vi "Target.vi"   [LabVIEW 2025]
uses:
  <vilib>/eio/utilities/niEioResolveVilibRelativePath.vi
  <vilib>/rvi/interface/RandomDataEmulation/niFpgaRandomDataHandleErrors.vi
  <vilib>/rvi/Memory/Memory_Emulation/nirvimemoryFastEmulation.vi
  <vilib>/rvi/Memory/Memory_Emulation/nirvimemoryEmulation.vi
  <vilib>/rvi/Emulation/niFpgaEmulationIsFPGAContextNoSignature.vi
  <vilib>/rvi/DataTransferAndStorage/Container/Common/niFpgaContainerGetUniqueNameForEmu.vi
  <vilib>/rvi/Emulation/niFpgaProcessEmulError.vi
  <vilib>/rvi/Emulation/niFpgaSctlEmulationGetInTimedLoop.vi
  <vilib>/rvi/errors/nirviReportUnexpectedCaseInternalError (U32).vi
  <vilib>/rvi/DataTransferAndStorage/Container/XNode/niFpgaContainer.xnode
  <vilib>/rvi/interface/RandomDataEmulation/nirviRandomDataFpgaReadWriteTemplate.vi
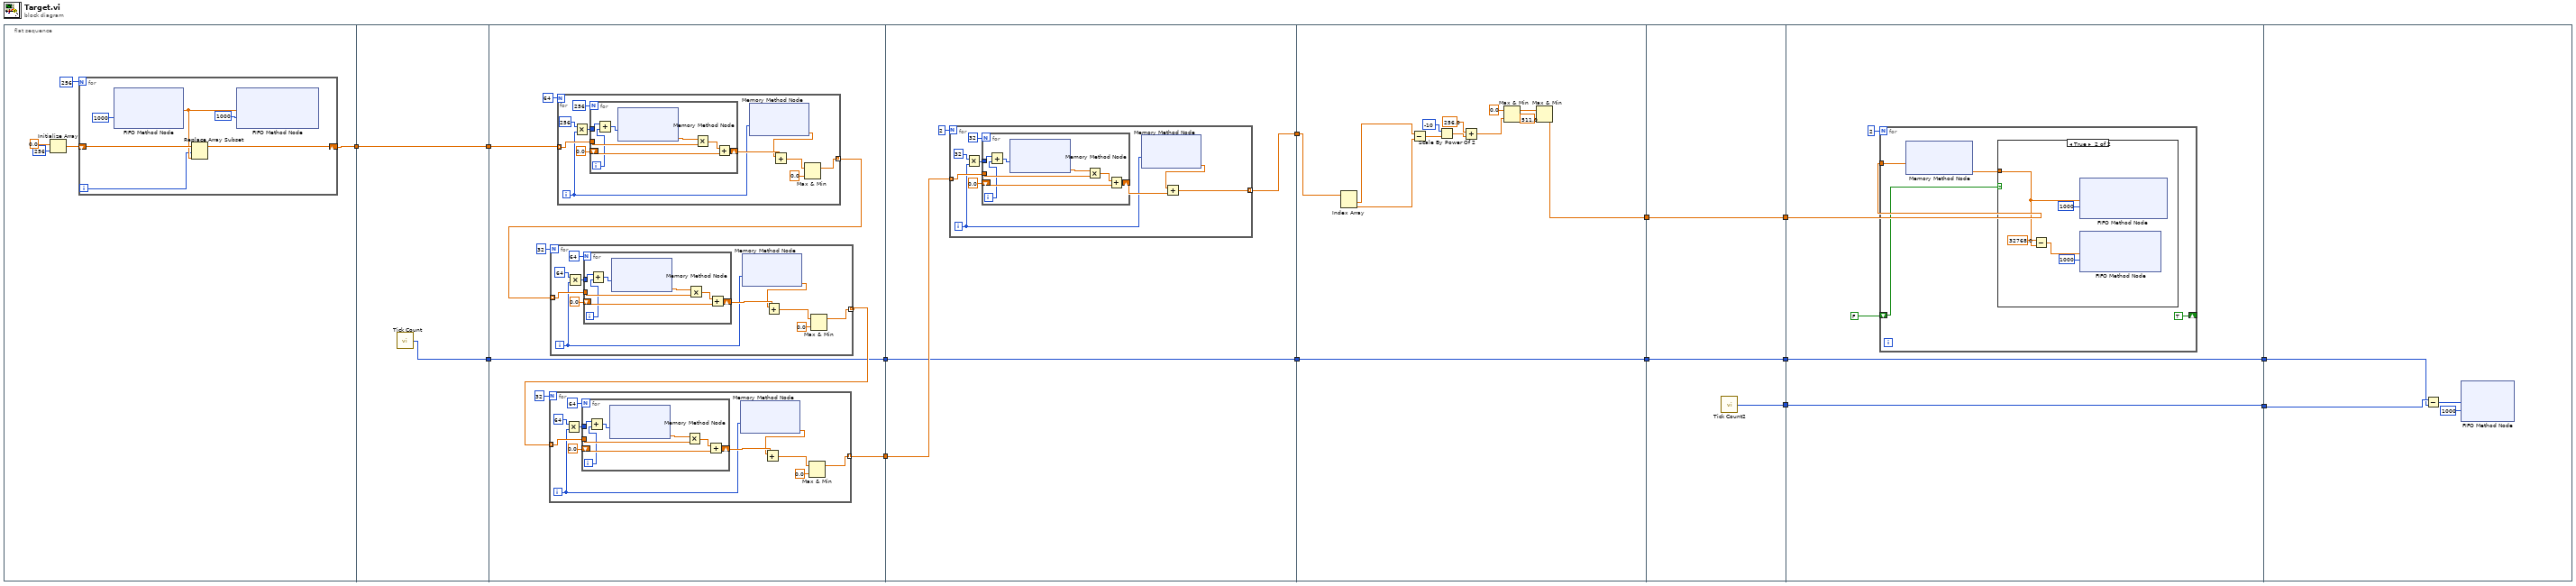
[diagram p0: block diagram]
diagram:
  n1 = flat-sequence {
    tunnel: [w18] -> w14
    tunnel: w14 -> [w27]
    tunnel: [w27] -> w13
    tunnel: [w26] -> w12
    tunnel: w13 -> [w30]
    tunnel: [w29] -> w11
    tunnel: w12 -> [w28]
    tunnel: [w28] -> w10
    tunnel: w11 -> [w95]
    tunnel: [w94] -> w9
    tunnel: w10 -> [w93]
    tunnel: [w93] -> w8
    tunnel: w9 -> [w116]
    tunnel: [w115] -> w7
    tunnel: w8 -> [w114]
    tunnel: [w114] -> w6
    tunnel: w7 -> [w129]
    tunnel: [w129] -> w5
    tunnel: w6 -> [w128]
    tunnel: [w128] -> w4
    tunnel: [w127] -> w3
    tunnel: w5 -> [w133]
    tunnel: [w130] -> w2
    tunnel: w4 -> [w131]
    tunnel: [w131] -> w1
    tunnel: w3 -> [w130]
    tunnel: w2 -> [w147]
    tunnel: w1 -> [w146]
    frame #0 {
      n2 = Initialize Array(sgl 0.0 ("element"), 256 ("dimension size")) -> (w15:sgl[])
      n3 = for {
        N: 256 -> [_]
        shift-right: [w21] -> w18
        shift-left: w15 -> [w23]
        i -> [w20]
        n4 = xnode ("FIFO Method Node")("Timeout"=1000) -> ("Element"=w22:sgl)  [unwired: 1 in, 2 out]
        n5 = Replace Array Subset(array=w23, new element=w22, index=w20) -> (w21:sgl[])
        n6 = xnode ("FIFO Method Node")("Element"=w22, "Timeout"=1000) -> ()  [unwired: 1 in, 2 out]
      }
    }
    frame #1 {
      n7 = call "Tick Count"() -> ("Tick Count(uSec)"=w26:u32)
    }
    frame #2 {
      n8 = for {
        N: 64 -> [_]
        tunnel: w30 -> [w84] mode=indexing
        tunnel: [w75] -> w34 mode=indexing
        i -> [w79]
        n9 = Multiply(x=256, y=w79) -> (x*y=w78:i32)
        n10 = for {
          N: 256 -> [_]
          tunnel: w84 -> [w90]
          shift-right: [w89] -> w82
          shift-left: sgl 0.0 -> [w88]
          tunnel: w78 -> [w87]
          i -> [w86]
          n11 = Add(x=w87, y=w86) -> (x+y=w85:i32)
          n12 = xnode ("Memory Method Node")("Address"=w85) -> ("Data"=w92:sgl)  [unwired: 1 in, 1 out]
          n13 = Multiply(x=w92, y=w90) -> (x*y=w91:sgl)
          n14 = Add(x=w91, y=w88) -> (x+y=w89:sgl)
        }
        n15 = xnode ("Memory Method Node")("Address"=w79) -> ("Data"=w81:sgl)  [unwired: 1 in, 1 out]
        n16 = Add(x=w81, y=w82) -> (x+y=w77:sgl)
        n17 = Max & Min(x=w77, y=sgl 0.0) -> (max(x,y)=w75:sgl)  [unwired: 1 out]
      }
      n18 = for {
        N: 32 -> [_]
        tunnel: w34 -> [w65] mode=indexing
        tunnel: [w56] -> w35 mode=indexing
        i -> [w60]
        n19 = Multiply(x=64, y=w60) -> (x*y=w59:i32)
        n20 = for {
          N: 64 -> [_]
          tunnel: w65 -> [w71]
          shift-right: [w70] -> w63
          shift-left: sgl 0.0 -> [w69]
          tunnel: w59 -> [w68]
          i -> [w67]
          n21 = Add(x=w68, y=w67) -> (x+y=w66:i32)
          n22 = xnode ("Memory Method Node")("Address"=w66) -> ("Data"=w73:sgl)  [unwired: 1 in, 1 out]
          n23 = Multiply(x=w73, y=w71) -> (x*y=w72:sgl)
          n24 = Add(x=w72, y=w69) -> (x+y=w70:sgl)
        }
        n25 = xnode ("Memory Method Node")("Address"=w60) -> ("Data"=w62:sgl)  [unwired: 1 in, 1 out]
        n26 = Add(x=w62, y=w63) -> (x+y=w57:sgl)
        n27 = Max & Min(x=w57, y=sgl 0.0) -> (max(x,y)=w56:sgl)  [unwired: 1 out]
      }
      n28 = for {
        N: 32 -> [_]
        tunnel: w35 -> [w46] mode=indexing
        tunnel: [w37] -> w29 mode=indexing
        i -> [w41]
        n29 = Multiply(x=64, y=w41) -> (x*y=w40:i32)
        n30 = for {
          N: 64 -> [_]
          tunnel: w46 -> [w52]
          shift-right: [w51] -> w44
          shift-left: sgl 0.0 -> [w50]
          tunnel: w40 -> [w49]
          i -> [w48]
          n31 = Add(x=w49, y=w48) -> (x+y=w47:i32)
          n32 = xnode ("Memory Method Node")("Address"=w47) -> ("Data"=w54:sgl)  [unwired: 1 in, 1 out]
          n33 = Multiply(x=w54, y=w52) -> (x*y=w53:sgl)
          n34 = Add(x=w53, y=w50) -> (x+y=w51:sgl)
        }
        n35 = xnode ("Memory Method Node")("Address"=w41) -> ("Data"=w43:sgl)  [unwired: 1 in, 1 out]
        n36 = Add(x=w43, y=w44) -> (x+y=w38:sgl)
        n37 = Max & Min(x=w38, y=sgl 0.0) -> (max(x,y)=w37:sgl)  [unwired: 1 out]
      }
    }
    frame #3 {
      n38 = for {
        N: 2 -> [_]
        tunnel: w95 -> [w105] mode=indexing
        tunnel: [w98] -> w94 mode=indexing
        i -> [w100]
        n39 = Multiply(x=32, y=w100) -> (x*y=w99:i32)
        n40 = for {
          N: 32 -> [_]
          tunnel: w105 -> [w111]
          shift-right: [w110] -> w103
          shift-left: sgl 0.0 -> [w109]
          tunnel: w99 -> [w108]
          i -> [w107]
          n41 = Add(x=w108, y=w107) -> (x+y=w106:i32)
          n42 = xnode ("Memory Method Node")("Address"=w106) -> ("Data"=w113:sgl)  [unwired: 1 in, 1 out]
          n43 = Multiply(x=w113, y=w111) -> (x*y=w112:sgl)
          n44 = Add(x=w112, y=w109) -> (x+y=w110:sgl)
        }
        n45 = xnode ("Memory Method Node")("Address"=w100) -> ("Data"=w102:sgl)  [unwired: 1 in, 1 out]
        n46 = Add(x=w102, y=w103) -> (x+y=w98:sgl)
      }
    }
    frame #4 {
      n47 = Index Array(array=w116) -> (element #1=w121:sgl, element #2=w122:sgl)  [unwired: 2 in]
      n48 = Subtract(x=w121, y=w122) -> (x-y=w123:sgl)
      n49 = Scale By Power Of 2(n=i16 -10, x=w123) -> (x*2^n=w124:sgl)
      n50 = Add(x=sgl 256.0, y=w124) -> (x+y=w125:sgl)
      n51 = Max & Min(x=sgl 0.0, y=w125) -> (max(x,y)=w126:sgl)  [unwired: 1 out]
      n52 = Max & Min(x=w126, y=sgl 511.0) -> (min(x,y)=w115:sgl)  [unwired: 1 out]
    }
    frame #5 {
      n53 = call "Tick Count2"() -> ("Tick Count(uSec)"=w127:u32)
    }
    frame #6 {
      n54 = for {
        N: 2 -> [_]
        tunnel: w133 -> [w138]
        shift-right: [TRUE] -> _
        shift-left: FALSE -> [w137]
        n55 = xnode ("Memory Method Node")("Address"=w138) -> ("Data"=w135:sgl)  [unwired: 1 in, 1 out]
        n56 = case shown="True" w137 {
          tunnel: w135 -> [_ w139]
          frame False {
          }
          frame True {
            n57 = Subtract(x=sgl 32768.0, y=w139) -> (x-y=w143:sgl)
            n58 = xnode ("FIFO Method Node")("Element"=w139, "Timeout"=1000) -> ()  [unwired: 1 in, 2 out]
            n59 = xnode ("FIFO Method Node")("Element"=w143, "Timeout"=1000) -> ()  [unwired: 1 in, 2 out]
          }
        }
      }
    }
    frame #7 {
      n60 = Subtract(x=w147, y=w146) -> (x-y=w145:u32)
      n61 = xnode ("FIFO Method Node")("Element"=w145, "Timeout"=1000) -> ()  [unwired: 1 in, 2 out]
    }
  }
